vi "Basic Generate LV Icon Text Layer.vi"(8 "error in (no error)":errorcluster, 10 "Text":T1={"Line 1 text"="", "Line 2 text"="a", "Line 3 text"="b", "Line 4 text"="c"}, 11 "Icon":refnum<class "Icon.lvclass">) -> (0 "error out":errorcluster, 3 "Icon.lvlclass out":refnum<class "Icon.lvclass">)   [LabVIEW 2019, in "gRPC Template Creation Utility.lvlib"]
doc: "Basic example that shows how to set the Text Layer"
uses:
  gRPC Template Creation Utility.lvlib
  <vilib>/LabVIEW Icon API/lv_icon/Classes/Icon/Icon.lvclass
  <vilib>/LabVIEW Icon API/API_Rectangle Dimension.ctl
  <vilib>/LabVIEW Icon API/API_Test Settings.ctl
  <vilib>/LabVIEW Icon API/lv_icon/Controls/Alignment.ctl
  <vilib>/LabVIEW Icon API/API_Text Colors.ctl
  <vilib>/LabVIEW Icon API/LabVIEW Icon API.lvlib
  <vilib>/LabVIEW Icon API/API_Text.ctl
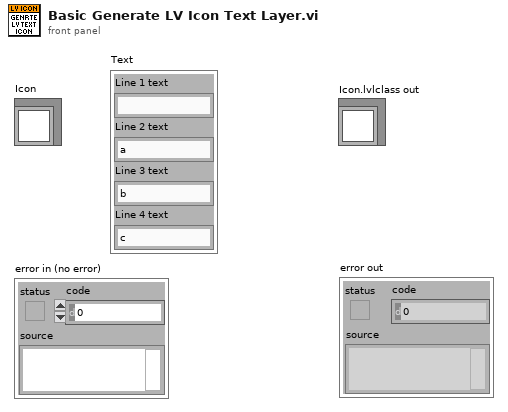
[diagram p1: front panel]
types:
  T1 = typedef "LabVIEW Icon API.lvlib/API_Text.ctl" = cluster{"Line 1 text":string, "Line 2 text":string, "Line 3 text":string, "Line 4 text":string}
  T2 = typedef "LabVIEW Icon API.lvlib/API_Test Settings.ctl" = cluster{"Font":string, "Alignment":T3, "Size":u8, "Center text":bool, "Capitalize text":bool, "Text color":T4}
  T3 = typedef "Alignment.ctl" = u16
  T4 = typedef "LabVIEW Icon API.lvlib/API_Text Colors.ctl" = cluster{"Line 1 color":u32, "Line 2 color":u32, "Line 3 color":u32, "Line 4 color":u32}
  T5 = typedef "LabVIEW Icon API.lvlib/API_Rectangle Dimension.ctl" = cluster{"Width":i16, "Height":i16}
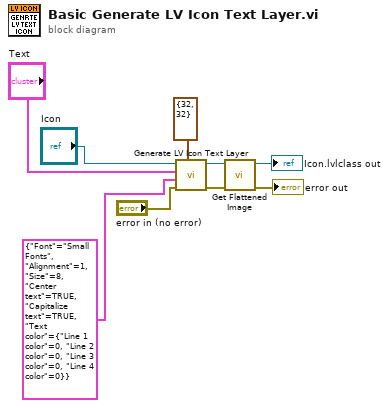
[diagram p0: block diagram]
diagram:
  n1 = call <vilib>:"Generate LV Icon Text Layer.vi"("Rectangle dimension (32,32)"=T5 {"Width"=32, "Height"=32}, "error in (no error)"="error in (no error)", "Text settings"=T2 {"Font"="Small Fonts", "Alignment"=1, "Size"=8, "Center text"=TRUE, "Capitalize text"=TRUE, "Text color"={"Line 1 color"=0, "Line 2 color"=0, "Line 3 color"=0, "Line 4 color"=0}}, "Text"="Text", "Icon in"="Icon") -> ("error out"=w3:errorcluster, "Icon out"=w4:refnum<class "Icon.lvclass">)  [unwired: 5 in]
  n2 = call <vilib>:"Get Flattened Image.vi"("error in (no error)"=w3, "lv_icon.lvlib:Icon.lvclass in"=w4) -> ("error out"=→"error out":errorcluster, "lv_icon.lvlib:Icon.lvclass out"=→"Icon.lvlclass out":refnum<class "Icon.lvclass">)  [unwired: 6 in, 2 out]
